vi "getDefault.vi"(9 "Numeric 2":dbl, 10 "defaults":string, 11 "value":string) -> (2 "value 2":string)   [LabVIEW 2014]
panel:
  out "default array":string[](array[string])
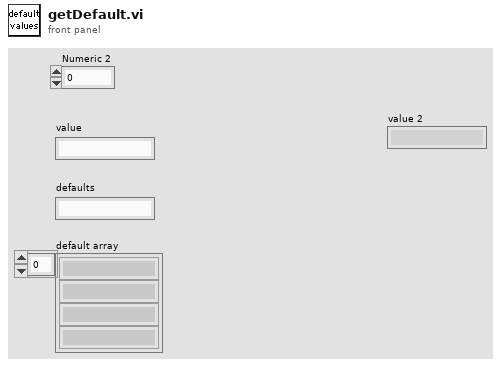
[diagram p1: front panel]
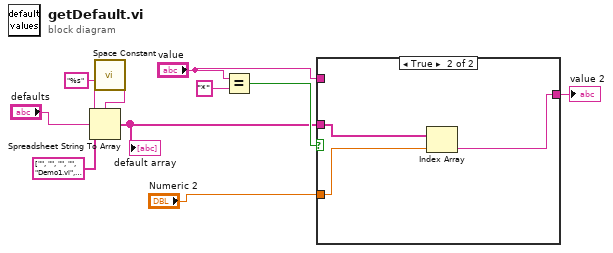
[diagram p0: block diagram]
diagram:
  n1 = call <vilib>:"Space Constant.vi"() -> ("String"=w2:string)
  n2 = Spreadsheet String To Array(delimiter (Tab)=w2, format string="%s", spreadsheet string="defaults", array type (2D Dbl)=string[] ["", "", "", "", "Demo1.vi", "DigitalWrite.vi", "VS_Wait.vi", ""] ("Array 3")) -> (array=w1:string[])
  "default array" <- w1
  n3 = Equal?(x="value", y="*") -> (x = y?=w9:bool)
  n4 = case shown="True" w9 {
    tunnel: "value" -> [w11 _]
    tunnel: "Numeric 2" -> [_ w13]
    tunnel: [w11 w12] -> w6
    tunnel: w1 -> [_ w14]
    frame False {
    }
    frame True {
      n5 = Index Array(array=w14, index=w13) -> (element=w12:string)
    }
  }
  "value 2" <- w6
